vi "Open Motors.vi"(0 "PID":cluster{"P":dbl, "I":dbl, "D":dbl}) -> (1 "Left Motor Refs":T1={"DeviceStatus"={"status"=FALSE, "code"=0, "source"=""}, "Type"=enum."PWM", "PWM"={"PWM Channel"=enum."PWM 1", "DeadBand"={"Name"="", "maxPositivePwm"=0, "minPositivePwm"=0, "centerPwm"=0, "maxNegativePwm"=0, "minNegativePwm"=0, "angularRange"=0}}, "CAN"={"Device Number"=0, "Control Mode"=enum."Percent VBus", "Semaphore"=refnum, "Max Vout"=12.0, "TalonSRX Control Mode"=enum."Percent VBus"}, "Invert"=FALSE}, 2 "Right Motor Refs":T1={"DeviceStatus"={"status"=FALSE, "code"=0, "source"=""}, "Type"=enum."PWM", "PWM"={"PWM Channel"=enum."PWM 1", "DeadBand"={"Name"="", "maxPositivePwm"=0, "minPositivePwm"=0, "centerPwm"=0, "maxNegativePwm"=0, "minNegativePwm"=0, "angularRange"=0}}, "CAN"={"Device Number"=0, "Control Mode"=enum."Percent VBus", "Semaphore"=refnum, "Max Vout"=12.0, "TalonSRX Control Mode"=enum."Percent VBus"}, "Invert"=FALSE})   [LabVIEW 2015]
uses:
  <vilib>/Rock Robotics/WPI/MotorControl/WPI_MotorControlDeviceRef.ctl
  <vilib>/Rock Robotics/WPI/MotorControl/WPI_MotorControlType.ctl
  <vilib>/Rock Robotics/SystemInterfaces/DIO/FPGA_DIOPWMChannel.ctl
  <vilib>/Rock Robotics/WPI/PWM/WPI_PWMDeadband.ctl
  <vilib>/Rock Robotics/WPI/CAN/Jaguar/SubVIs/WPI_CANJaguar_ControlMode.ctl
  <vilib>/Rock Robotics/WPI/CAN/TalonSRX/WPI_CANTalonSRX_APIControlMode.ctl
  <vilib>/Rock Robotics/WPI/MotorControl/WPI_MotorControlOpenCANTalonSRX.vi
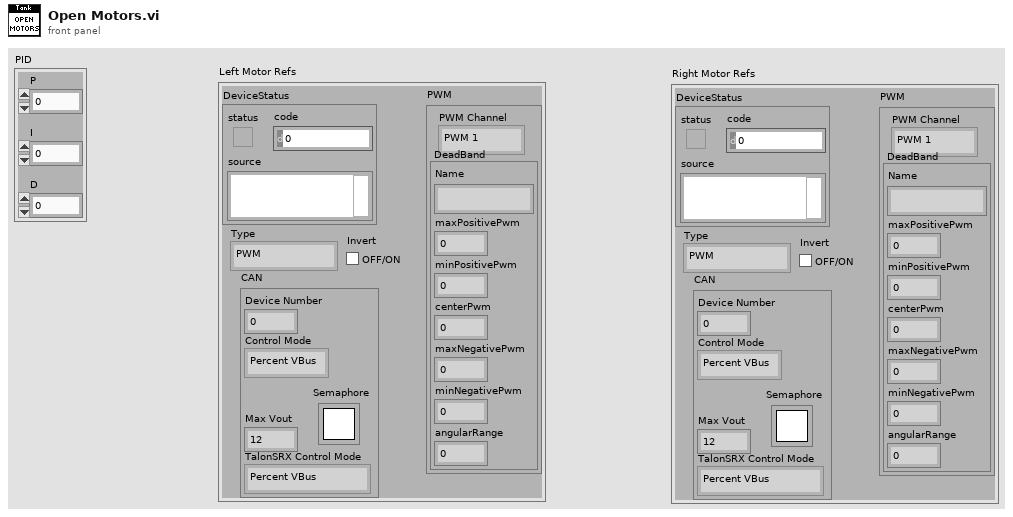
[diagram p1: front panel]
types:
  T1 = typedef "WPI_MotorControlDeviceRef.ctl" = cluster{"DeviceStatus":errorcluster, "Type":T2, "PWM":cluster{"PWM Channel":T3, "DeadBand":T4}, "CAN":cluster{"Device Number":u8, "Control Mode":T5, "Semaphore":T6, "Max Vout":dbl, "TalonSRX Control Mode":T7}, "Invert":bool}
  T2 = typedef "WPI_MotorControlType.ctl" = enum16{"PWM", "CAN", "CANTalonSRX"}
  T3 = typedef "FPGA_DIOPWMChannel.ctl" = enum8{"PWM 0", "PWM 1", "PWM 2", "PWM 3", "PWM 4", "PWM 5", "PWM 6", "PWM 7", "PWM 8", "PWM 9", "PWM MXP 0", "PWM MXP 1", "PWM MXP 2", "PWM MXP 3", "PWM MXP 4", "PWM MXP 5", "PWM MXP 6", "PWM MXP 7", "PWM MXP 8", "PWM MXP 9", "Invalid"}
  T4 = typedef "WPI_PWMDeadband.ctl" = cluster{"Name":string, "maxPositivePwm":i32, "minPositivePwm":i32, "centerPwm":i32, "maxNegativePwm":i32, "minNegativePwm":i32, "angularRange":u16}
  T5 = typedef "WPI_CANJaguar_ControlMode.ctl" = enum8{"Percent VBus", "Current", "Speed", "Position", "Voltage"}
  T6 = typedef "Semaphore RefNum" = refnum<k1>
  T7 = typedef "WPI_CANTalonSRX_APIControlMode.ctl" = enum8{"Percent VBus", "Speed", "Position", "Slave", "Unchanged / Invalid", "Voltage Compensation", "Current", "Motion Profile"}
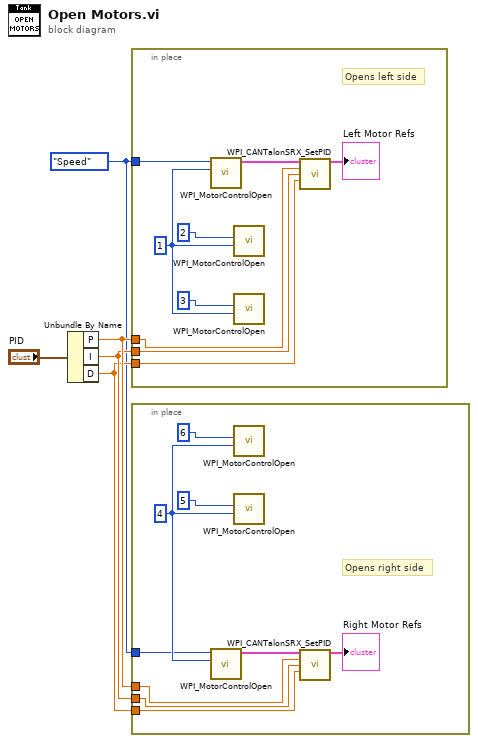
[diagram p0: block diagram]
diagram:
  w1 = WPI_CANTalonSRX_APIControlMode."Speed" ("Control Mode")
  n1 = Unbundle By Name("PID") -> ("P"=w4:dbl, "I"=w3:dbl, "D"=w2:dbl)
  n2 = in-place {
    in-place-border: w1 -> [w11]
    in-place-border: w4 -> [w9]
    in-place-border: w3 -> [w8]
    in-place-border: w2 -> [w7]
    w12 = u8 1 ("Device Number")
    # "Opens left side"
    n3 = call-poly <vilib>:"WPI_MotorControlOpen.vi"("Device Number"=w12, "Control Mode"=w11) -> ("MotorControlDeviceRef"=w10:T1)  [unwired: 8 in, 1 out]
    n4 = call-poly <vilib>:"WPI_MotorControlOpen.vi"("Master Device Number"=w12, "Device Number"=u8 2) -> ()  [unwired: 8 in, 2 out]
    n5 = call-poly <vilib>:"WPI_MotorControlOpen.vi"("Master Device Number"=w12, "Device Number"=u8 3) -> ()  [unwired: 8 in, 2 out]
    n6 = call <vilib>:"WPI_CANTalonSRX_SetPID.vi"("CAN Talon SRX Ref"=w10, "P"=w9, "I"=w8, "D"=w7) -> ("CAN Talon SRX Ref"=→"Left Motor Refs":T1)  [unwired: 10 in, 1 out]
  }
  n7 = in-place {
    in-place-border: w4 -> [w19]
    in-place-border: w3 -> [w18]
    in-place-border: w2 -> [w17]
    in-place-border: w1 -> [w15]
    w20 = u8 4 ("Device Number")
    # "Opens right side"
    n8 = call-poly <vilib>:"WPI_MotorControlOpen.vi"("Device Number"=w20, "Control Mode"=w15) -> ("MotorControlDeviceRef"=w23:T1)  [unwired: 8 in, 1 out]
    n9 = call-poly <vilib>:"WPI_MotorControlOpen.vi"("Master Device Number"=w20, "Device Number"=u8 6) -> ()  [unwired: 8 in, 2 out]
    n10 = call-poly <vilib>:"WPI_MotorControlOpen.vi"("Master Device Number"=w20, "Device Number"=u8 5) -> ()  [unwired: 8 in, 2 out]
    n11 = call <vilib>:"WPI_CANTalonSRX_SetPID.vi"("CAN Talon SRX Ref"=w23, "P"=w19, "I"=w18, "D"=w17) -> ("CAN Talon SRX Ref"=→"Right Motor Refs":T1)  [unwired: 10 in, 1 out]
  }
